vi "LQR.vi"() -> ()   [LabVIEW 2021]
uses:
  <vilib>/addons/Control Design/_Model Construction/Model Typedefs.llb/CD State Space Model (MIMO).ctl
  <vilib>/addons/Control Design/_Model Construction/Model Typedefs.llb/CD General Elements.ctl
  <vilib>/Analysis/Matrix/Datatypes/RealMatrix.ctl
  <vilib>/Simulation/Scripting/Companion Diagram/SimConfigNode/SimParams.ctl
  <vilib>/Simulation/Scripting/Companion Diagram/SimConfigNode/_simSolvers.ctl
  <vilib>/Simulation/Implementation/Shared/SIMSCR Execution Mode.ctl
  <vilib>/Simulation/Param Hierarchy/Typedefs/SIMPH Param Control Actions.ctl
  <vilib>/Simulation/Implementation/Shared/NILVSim_ParamChanged.vi
  <vilib>/Simulation/Implementation/Shared/NILVSIM_BeginStep.vi
  <vilib>/Simulation/DataSources/Implementation/NILVSim Step.llb/SIM Step (scalar).vi
  <vilib>/Simulation/ContinuousLinear/Implementation/NILVSim State Space.llb/SIM State Space Distributor (CD).vi
  <vilib>/Simulation/SignalDisplay/Implementation/NILVSim Time Waveform.llb/SIM Time Waveform (vector).vi
  <vilib>/Simulation/SignalArithmetic/Implementation/NILVSim Gain.llb/SIM Gain (vector,MatrixGain).vi
  <vilib>/Simulation/SignalArithmetic/Implementation/NILVSim Gain.llb/SIM Gain (vector,ScalarGain).vi
  <vilib>/Simulation/ContinuousLinear/Implementation/NILVSim State Space.llb/SIM State Space Collector (CD).vi
  <vilib>/Simulation/Implementation/Shared/NILVSim_Manager.vi
  <vilib>/Utility/error.llb/Clear Errors.vi
  <vilib>/Simulation/Implementation/Shared/NILVSim_FinalizeModel.vi
  <vilib>/addons/Control Design/_Model Construction/Model Creation.llb/Model Creation SubVI/cd_Create State Space Model.vi
  <vilib>/addons/Control Design/_Dynamic Analysis/Dynamic Analysis.llb/Dynamic Analysis subVI/cd_Poles (State-Space).vi
  <vilib>/addons/Control Design/_Utility/Model Viewer.llb/Model Viewer SubVI/cd_Draw State-Space Equation (SS).vi
  <vilib>/Analysis/baseanly.llb/Real Inverse Matrix.vi
  <vilib>/addons/Control Design/_State Feedback Control/State Feedback Control.llb/State Feedback Control SubVis/cd_Linear Quadratic Regulator.vi
  <vilib>/Simulation/Implementation/Shared/SIM Unbundle Sim Info.vi
  <vilib>/Simulation/Implementation/Shared/NILVSim_Initialize.vi
  <vilib>/Simulation/Utility/Implementation/NILVSim Get Time and IsAcceptedStep.vi
  <vilib>/Simulation/Implementation/Shared/SIMSH Read Queue.vi
  <vilib>/Simulation/Implementation/Shared/NILVSim_GetModelError.vi
  <vilib>/Simulation/Implementation/Shared/SIM Bundle Sim Info.vi
  <vilib>/Simulation/Scripting/Companion Diagram/SimConfigNode/SimDog.xnode
  <vilib>/Simulation/Implementation/XNodeFramework/SimXNode/SimX.xnode
  <vilib>/addons/Control Design/_Model Construction/NI_LinSys_Model Creation.lvlib
  <vilib>/addons/Control Design/_State-Space Analysis/NI_CD_State-Space Analysis.lvlib
  <vilib>/addons/Control Design/_Utility/NI_CD_Model Viewer.lvlib
  <vilib>/Analysis/NI_AALBase.lvlib
  <vilib>/addons/Control Design/_Dynamic Analysis/NI_CD_Dynamic Analysis.lvlib
  <vilib>/addons/Control Design/_Model Construction/NI_LinSys_Model Typedefs.lvlib
  <vilib>/addons/Control Design/_State Feedback Control/NI_CD_State Feedback Control.lvlib
  <vilib>/Simulation/ContinuousLinear/Implementation/NILVSim State Space.llb/SIM State Space (CD).vi
  <vilib>/Simulation/Implementation/Shared/NI_SIM_Implementation.lvlib
  <vilib>/Analysis/Matrix/NI_Matrix.lvlib
panel:
  out "Waveform Chart 5":waveform(dbl)[](graph)=[{"t0"=timestamp(10 s since 1904-01-01), "dt"=1.0, "Y"=[0.10162173161595328]}, {"t0"=timestamp(10 s since 1904-01-01), "dt"=1.0, "Y"=[-2.6765462739759283e-05]}, {"t0"=timestamp(10 s since 1904-01-01), "dt"=1.0, "Y"=[-0.00047765810654039743]}, {"t0"=timestamp(10 s since 1904-01-01), "dt"=1.0, "Y"=[4.8571343408734025e-05]}]
  out "Waveform Chart 4":waveform(dbl)[](graph)=[{"t0"=timestamp(10 s since 1904-01-01), "dt"=1.0, "Y"=[0.10162173161595328]}, {"t0"=timestamp(10 s since 1904-01-01), "dt"=1.0, "Y"=[0.1]}]
  out "Riccati Solution (P)":dbl[][](array[numeric])=[[2.874895006147238, 15.790191536836533, 3.6325106481851583, 4.506008518548117], [15.790191536836533, 447.788780796216, 40.88913427681152, 124.16507438499208], [3.6325106481851583, 40.88913427681152, 8.831842687873085, 11.66530616013401], [4.506008518548117, 124.16507438499208, 11.66530616013401, 34.5965513870456]] format="%.2f"
  out "Eigenvalues":cdb[](array[numeric])=[-0.5280411546831855+0.4179135922160171i, -0.5280411546831855-0.4179135922160171i, -3.9913591922761484+0.0i, -3.3839807058066844+0.0i] format="%.2f"
  out "Control Action":waveform(dbl)[](graph)=[{"t0"=timestamp(10 s since 1904-01-01), "dt"=1.0, "Y"=[-0.0005144109686059197]}]
  out "Optimal Gain (K)":dbl[][](array[numeric])=[[-0.9999999999999939, -57.15860435221429, -2.874895006147214, -15.790191536836495]] format="%.2f"
  in  "R":dbl[][](array[numeric])=[[1.0]] format="%.2f"
  in  "Q":dbl[][](array[numeric])=[[1.0, 0.0, 0.0, 0.0], [0.0, 1.0, 0.0, 0.0], [0.0, 0.0, 1.0, 0.0], [0.0, 0.0, 0.0, 1.0]] format="%.2f"
  out "[0, K2, K3.....]":dbl[][](array[numeric])=[[0.0, -57.15860435221429, -2.874895006147214, -15.790191536836495]]
  out "K1":dbl=-0.9999999999999939
  in  "final value":dbl(slide)=0.1 scale=0.0..10.0
  out "Open Loop poles":cdb[](array[numeric])=[3.6708309685955305+0.0i, -3.67083096859553+0.0i, 0.0+0.0i, 0.0+0.0i] format="%.3f"
  out "T (transforamtion matrix)":T1=[[-6.125000000000001, -2.220446049250313e-16, 0.5, 1.7765721119653683e-33], [1.3288986138578397e-47, 2.7755575615628914e-16, -0.625, -2.2207151399567104e-33], [-2.7200464103316367e-16, -6.125000000000001, -2.2204460492503128e-16, 0.5], [3.740063814205997e-15, 0.0, 2.7755575615628914e-16, -0.625]]
  out "Equation":picture
  out "Transformation Matrix inverse(T-1)":dbl[][](array[numeric])=[[-0.16326530612244897, -0.13061224489795917, 0.0, 0.0], [-7.250436079184695e-17, -5.800348863347757e-17, -0.16326530612244897, -0.13061224489795917], [-3.2198404294735173e-32, -1.6, -7.250436079184695e-17, -5.800348863347756e-17], [-9.769962616701378e-16, -1.4921397450962105e-15, -3.2198404294735173e-32, -1.6]] format="%.2f"
  out "Transformed Model":T2={"properties"={"Model name"="System Model", "Input names"=["u0"], "Output names"=["y0"], "Input Delays"=[0.0], "Output Delays"=[0.0], "Sampling Time"=0.0, "Notes"=""}, "A"=[[-4.4408920985006257e-16, 0.9999999999999999, 1.5407439555097887e-33, -3.469446951953614e-18], [-1.9721522630525295e-31, 5.7777898331617076e-34, 0.9999999999999999, 6.162975822039155e-33], [-5.984102102729594e-15, 2.565854121688508e-49, -9.918539213594265e-32, 1.0], [-5.3149503489265676e-30, 2.98904327368899e-31, 13.475000000000001, 4.440892098500626e-16]], "B"=[[0.0], [-3.469446951953614e-18], [-1.5407439555097887e-33], [1.0]], "C"=[[-6.125, -2.220446049250313e-16, 0.5, 0.0]], "D"=[[0.0]], "StateNames"=["x0", "x1", "x2", "x3"], "Transport Delay"=[[0.0]]} {"Transport Delay" format="%.2f"; "D" format="%#.2g"; "C" format="%#.2g"; "B" format="%#.2g"; "A" format="%#.2g"; "properties"."Sampling Time" format="%#.6p"; "properties"."Output Delays" format="%.4f"; "properties"."Input Delays" format="%.4f"}
  in  "Form Type":u16(ring)=1 items=["Modal"=0, "Companion"=5, "Controllability"=1, "Controller Companion"=2, "Observability"=3, "Observer Companion"=4]
  out "Is Controllable?":bool=TRUE
  out "M (Controllability Matrix)":dbl[][](array[numeric])=[[0.0, 0.5, 0.0, 0.6125], [0.0, -0.625, 0.0, -8.421875], [0.5, 0.0, 0.6125, 0.0], [-0.625, 0.0, -8.421875, 0.0]] format="%.2f"
  in  "D":dbl[][](array[numeric])=[[0.0]] format="%#.5g"
  in  "C":dbl[][](array[numeric])=[[1.0, 0.0, 0.0, 0.0]] format="%#.5g"
  in  "B":dbl[][](array[numeric])=[[0.0], [0.0], [0.5], [-0.625]] format="%#.5g"
  in  "A":dbl[][](array[numeric])=[[0.0, 0.0, 1.0, 0.0], [0.0, 0.0, 0.0, 1.0], [0.0, -0.98, 0.0, 0.0], [0.0, 13.475, 0.0, 0.0]] format="%#.5g"
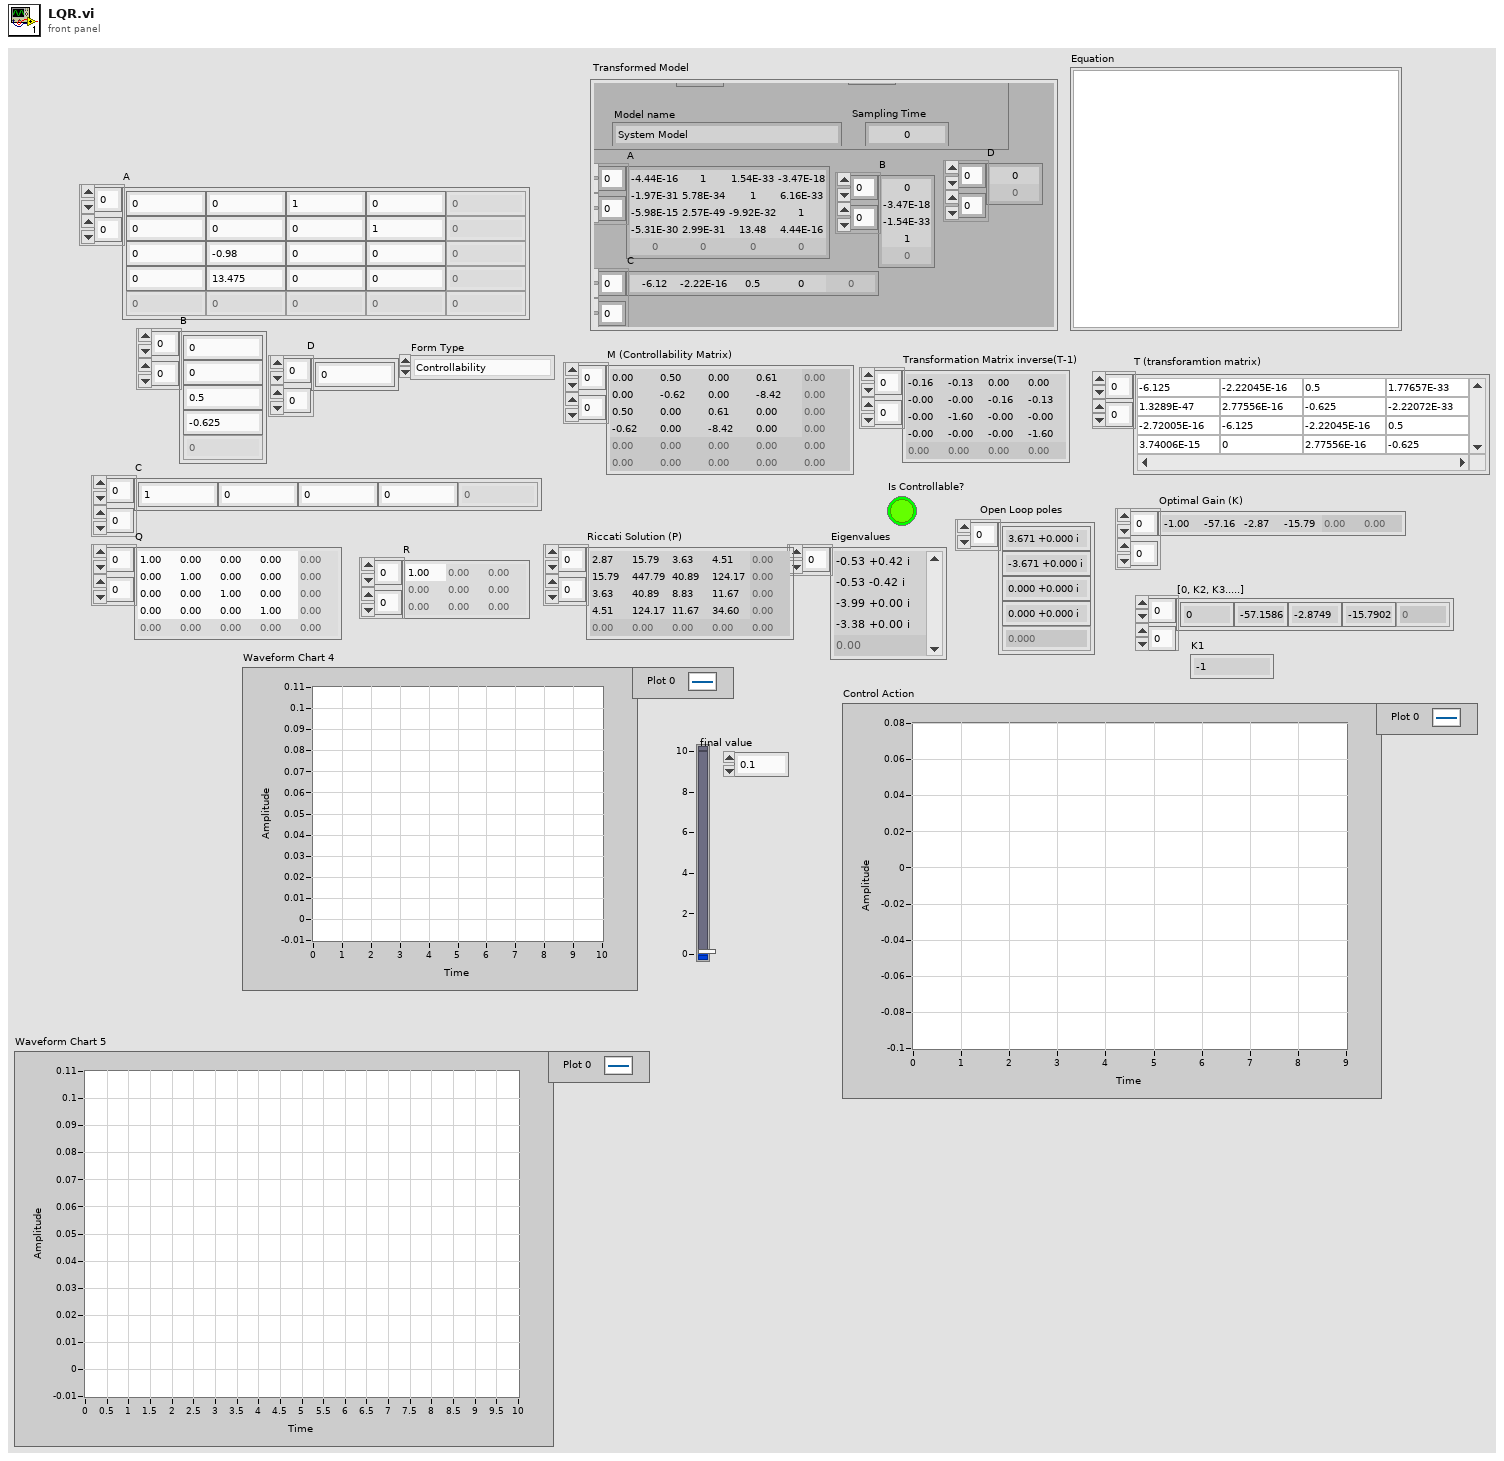
[diagram p1: front panel]
types:
  T1 = typedef "NI_Matrix.lvlib/RealMatrix.ctl" = dbl[][]
  T2 = typedef "NI_LinSys_Model Typedefs.lvlib/CD State Space Model (MIMO).ctl" = cluster{"properties":T3, "A":dbl[][], "B":dbl[][], "C":dbl[][], "D":dbl[][], "StateNames":string[], "Transport Delay":dbl[][]}
  T3 = typedef "NI_LinSys_Model Typedefs.lvlib/CD General Elements.ctl" = cluster{"Model name":string, "Input names":string[], "Output names":string[], "Input Delays":dbl[], "Output Delays":dbl[], "Sampling Time":dbl, "Notes":string}
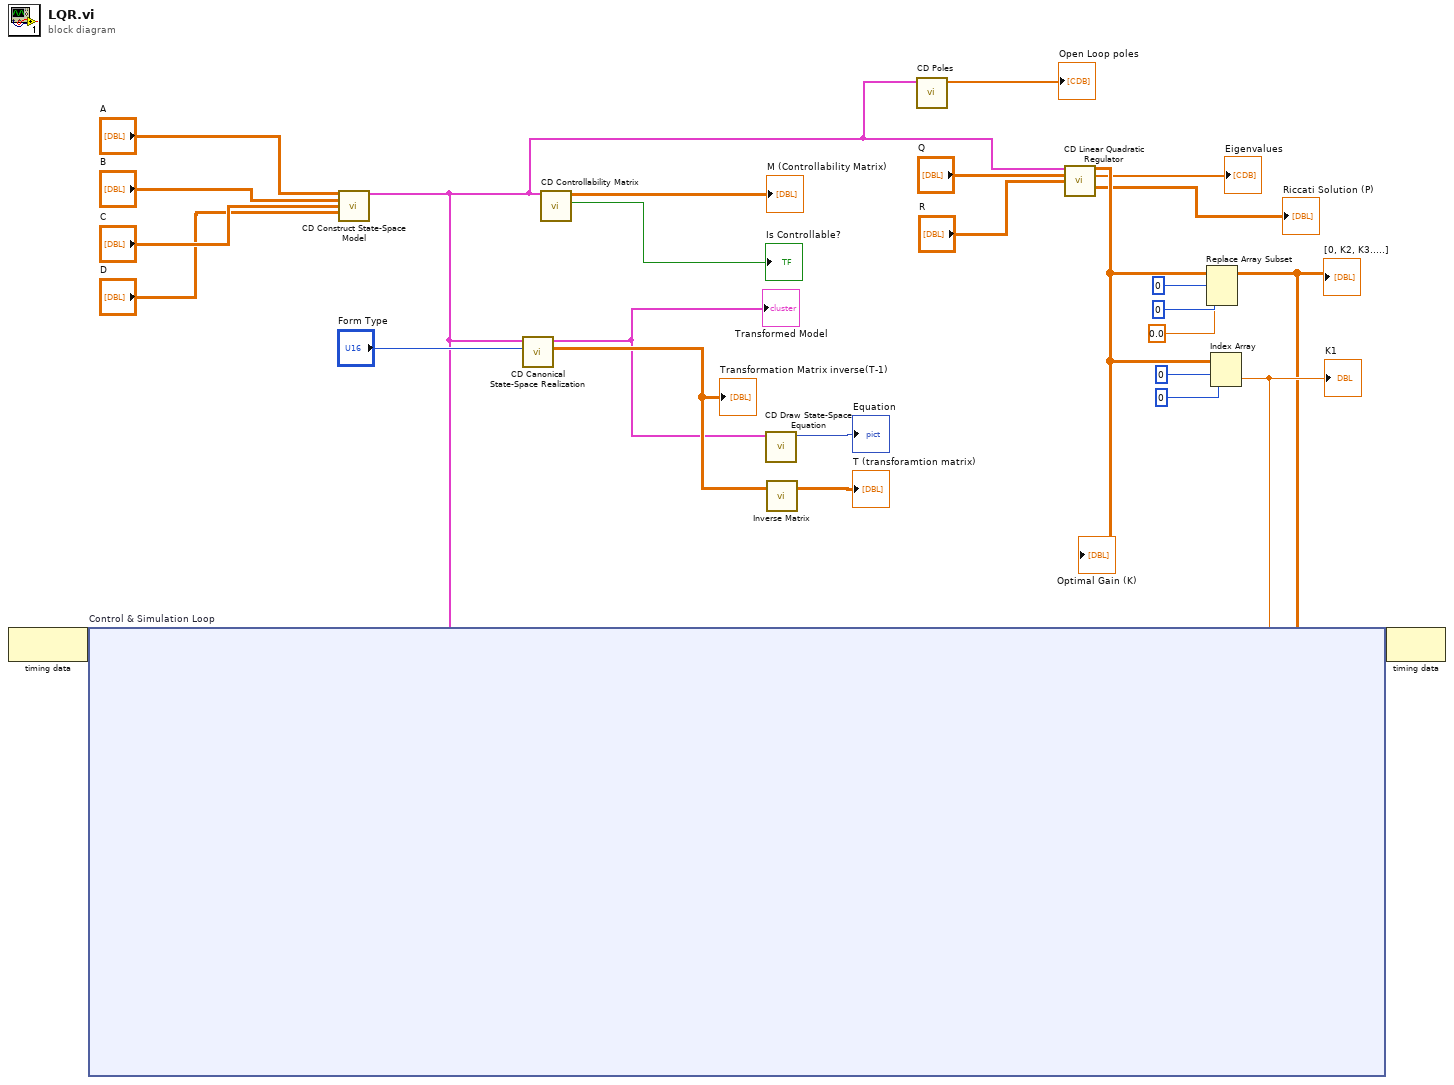
[diagram p0: block diagram]
diagram:
  n1 = node-c288() -> (w15:variant)  [unwired: 1 in]
  n2 = call-poly <vilib>:"CD Construct State-Space Model.vi"("A"="A", "B"="B", "C"="C", "D"="D") -> ("State-Space Model"=w4:T2)  [unwired: 10 in, 1 out]
  n3 = call <vilib>:"CD Canonical State-Space Realization.vi"("Form Type"="Form Type", "State-Space Model"=w4) -> ("Transformation Matrix (T)"=w23:dbl[][], "Transformed Model"=w16:T2)  [unwired: 7 in, 1 out]
  "Transformed Model" <- w16
  "Transformation Matrix inverse(T-1)" <- w23
  n4 = call <vilib>:"CD Controllability Matrix.vi"("State-Space Model"=w4) -> ("Is Controllable?"=→"Is Controllable?":bool, "Controllability Matrix"=→"M (Controllability Matrix)":dbl[][])  [unwired: 7 in, 2 out]
  n5 = call-poly <vilib>:"CD Draw State-Space Equation.vi"("State-Space Model"=w16) -> ("Equation"=→"Equation":picture)  [unwired: 8 in, 2 out]
  n6 = call-poly <vilib>:"Inverse Matrix.vi"("Input Matrix"=w23) -> ("Inverse Matrix"=→"T (transforamtion matrix)":T1)  [unwired: 1 in, 1 out]
  n7 = call-poly <vilib>:"CD Poles.vi"("State-Space Model"=w4) -> ("Poles"=→"Open Loop poles":cdb[])  [unwired: 9 in, 1 out]
  n8 = call-poly <vilib>:"CD Linear Quadratic Regulator.vi"("State-Space Model"=w4, "Q"="Q", "R"="R") -> ("Optimal Gain (K)"=w3:dbl[][], "Eigenvalues"=→"Eigenvalues":cdb[], "Riccati Solution (X)"=→"Riccati Solution (P)":dbl[][])  [unwired: 9 in, 1 out]
  "Optimal Gain (K)" <- w3
  n9 = Replace Array Subset(array=w3, new element=0.0 ("new element/subarray"), index (row)=0, index (col)=0 ("disabled index (col)")) -> (w7:dbl[][])
  "[0, K2, K3.....]" <- w7
  n10 = Index Array(array=w3, index (row)=0, index (col)=0 ("disabled index (col)")) -> (element=w11:dbl)
  "K1" <- w11
  n11 = node-c254 "Control & Simulation Loop"(w15, w4, w11, w7) -> (w14:variant)
  n12 = node-c288(w14) -> ()  [unwired: 1 out]
